vi "Write tsignal and tsensor elements u bazu_Core.vi"(9 "System_settings IN":T1={"Units in the system"=[], "dBase names by units"=[], "TCP/IP processing units addresses"=[], "TCP/IP server address"="", "dBase User Name_Cli"="codis_cli", "dBase User Password_Cli"="codis_cli", "dBase User Name_Med"="codis_med_wrt", "dBase User Password_Med"="codis_med_wrt", "Sampling rate [Hz]"=0.0, "FTP Server User name, cRIO"="", "FTP Server Password, cRIO"="", "OnScreenKeyboardPopUp"=FALSE, "Number of points to collect"=0, "Main Window has title bar?"=FALSE, "Demo?"=FALSE, "dBase - Limit # of  elements to read"=0, "dBase Backup"={"dBase Backup Base Folder"="c:\\codis\\backup\\", "Remote dBase Backup Configured?"=TRUE}, "System Status"={"System Monitor Refresh Rate (ms)"=10000, "System Status Log  File"="c:\\codis\\system_info.txt", "Max number of elements to read\n"=26611200}, "Number of points to average for stationary state"=[60], "Number of points to collect for saving waveforms per channel"=[60], "Sources per Unit"=[], "TCP/IP_client_mediator_communication ports"=2058, "TCP/IP processing_units _mediator_communication ports"=2055}, 10 "1D array of Pan Cluster IN":T10[](array[typedef]) {"Absolute Minimum Air Gap per Plane"."Absolute AG Minimum Pole Number" format="%.3f"; "Absolute Minimum Air Gap per Plane"."Absolute AG Minimum Value" format="%.3f"; "Magnetic Field Data"."Maximum by Pole Number" format="%.3f"; "Air Gap Data"."Minimum by Pole Number" format="%.3f"; "Orbit(s) - XY"."Orbit XY Graphs (Synthesized from Selected Harmonics and DC)"."?" format="%.3f"; "Orbit(s) - XY"."Orbit XY Graphs (Synthesized from Selected Harmonics and DC)"."?" format="%.3f"; "Orbit(s) - XY"."Orbit XY Graphs (Glided and Averaged on One Revolution)"."?" format="%.3f"; "Orbit(s) - XY"."Orbit XY Graphs (Glided and Averaged on One Revolution)"."?" format="%.3f"; "Orbit(s) - XY"."Orbit XY Graphs (Unaveraged)"."?" format="%.3f"; "Orbit(s) - XY"."Orbit XY Graphs (Unaveraged)"."?" format="%.3f"}, 11 "1D array of Waveform Cluster IN":T4[](array[typedef]) {"Analysis Parameters"."SP2Pmax"."Filter Parameters"."low cutoff freq: fl" format="%0.4f"; "Analysis Parameters"."SP2Pmax"."Filter Parameters"."high cutoff freq: fh" format="%0.2f"; "Analysis Parameters"."LoadAngleDelta"."Multiplication Factor" format="%.1f"; "Analysis Parameters"."LoadAngleDelta"."What harmonic? (for example 24th (48 pole machine))" format="%.1f"; "Analysis Parameters"."Peak2Peak"."Filter Parameters"."low cutoff freq: fl" format="%0.4f"; "Analysis Parameters"."Peak2Peak"."Filter Parameters"."high cutoff freq: fh" format="%0.2f"; "Analysis Parameters"."RMS"."Filter Parameters"."order" format="%0.4f"; "Analysis Parameters"."RMS"."Filter Parameters"."low cutoff freq: fl" format="%0.2f"; "Analysis Parameters"."RMS"."Filter Parameters"."high cutoff freq: fh" format="%0.2f"; "Analysis Parameters"."EqPeak"."Filter Parameters"."low cutoff freq: fl" format="%0.4f"; "Analysis Parameters"."EqPeak"."Filter Parameters"."high cutoff freq: fh" format="%0.2f"; "Analysis Parameters"."Peak"."Filter Parameters"."low cutoff freq: fl" format="%0.4f"; "Analysis Parameters"."Peak"."Filter Parameters"."high cutoff freq: fh" format="%0.2f"; "Analysis Parameters"."snPh"."What harmonic?" format="%.1f"; "Analysis Parameters"."snA"."Multiplication Factor" format="%.1f"; "Analysis Parameters"."snA"."What harmonic?" format="%.1f"; "Analysis Parameters"."Smax"."Filter Parameters"."low cutoff freq: fl" format="%0.4f"; "Analysis Parameters"."Smax"."Filter Parameters"."high cutoff freq: fh" format="%0.2f"; "Analysis Parameters"."RPM"."Signal Threshold" format="%.1f"}) -> (0 "error  OUT":errorcluster)   [LabVIEW 2014]
uses:
  common/typedefs/Pan_Cluster_Core.ctl
  common/typedefs/Condition_Vector_Cluster_Core.ctl
  common/typedefs/Unit_Names_Core.ctl
  common/typedefs/Data_Sources_Core.ctl
  common/typedefs/Waveforms_Cluster_Core.ctl
  common/typedefs/Types_of_Signals_Core.ctl
  common/typedefs/Types_of_Analyses_Core.ctl
  common/typedefs/Analysis_Parameters_Cluster_Core.ctl
  <vilib>/Analysis/3filter.llb/Filter Passband Type.ctl
  common/typedefs/Integration_Types_Core.ctl
  common/typedefs/System_Settings_Cluster_Client_Mediator_Core.ctl
  <vilib>/addons/database/Connection.llb/DB Tools Open Connec (String).vi
  <vilib>/addons/database/NI_Database_API.lvlib
  <vilib>/Analysis/NI_AALBase.lvlib
panel:
  out "error out 2":errorcluster
  out "error out":errorcluster
  out "Condition Vector Name":string[](array[string])
  out "Condition Vector Label":string[](array[string])
  out "Waveform Name":string[](array[string])
  out "Waveform Label":string[](array[string])
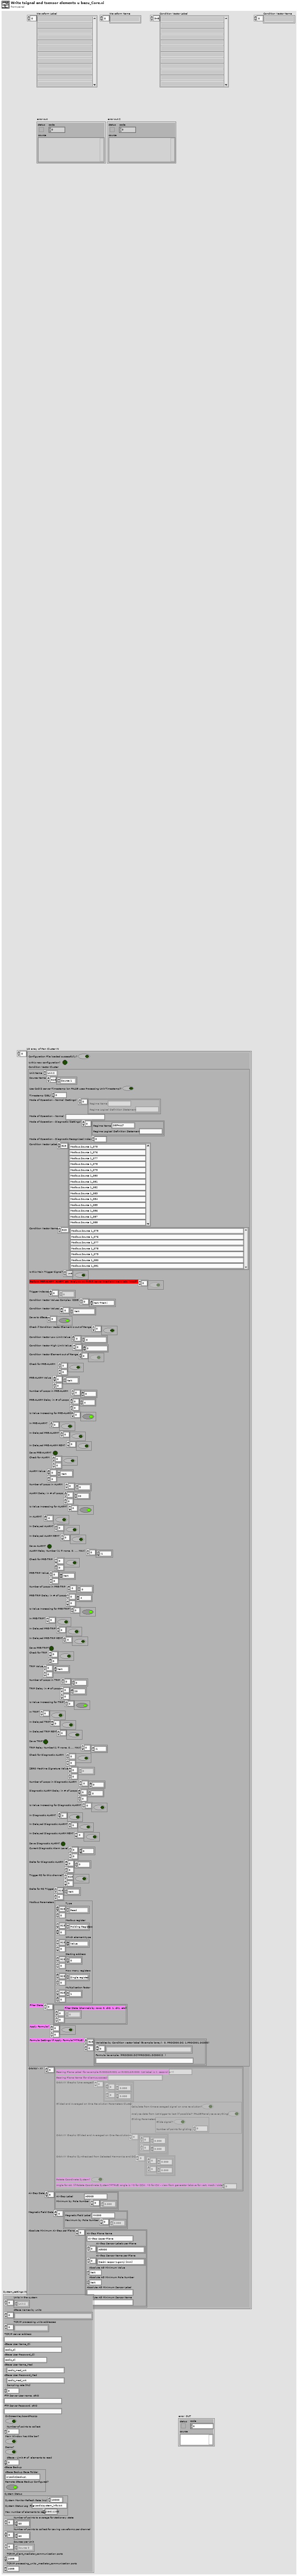
[diagram p1: front panel]
types:
  T1 = typedef "System_Settings_Cluster_Client_Mediator_Core.ctl" = cluster{"Units in the system":T2[], "dBase names by units":string[], "TCP/IP processing units addresses":string[], "TCP/IP server address":string, "dBase User Name_Cli":string, "dBase User Password_Cli":string, "dBase User Name_Med":string, "dBase User Password_Med":string, "Sampling rate [Hz]":dbl, "FTP Server User name, cRIO":string, "FTP Server Password, cRIO":string, "OnScreenKeyboardPopUp":bool, "Number of points to collect":u32, "Main Window has title bar?":bool, "Demo?":bool, "dBase - Limit # of  elements to read":u32, "dBase Backup":cluster{"dBase Backup Base Folder":string, "Remote dBase Backup Configured?":bool}, "System Status":cluster{"System Monitor Refresh Rate (ms)":u32, "System Status Log  File":string, "Max number of elements to read\n":i64}, "Number of points to average for stationary state":i32[], "Number of points to collect for saving waveforms per channel":i32[], "Sources per Unit":T3[], "TCP/IP_client_mediator_communication ports":u16, "TCP/IP processing_units _mediator_communication ports":u16}
  T2 = typedef "Unit_Names_Core.ctl" = enum16{"Not used", "Unit 1", "Unit 2", "Unit 3", "Unit 4", "Unit 5", "Unit 6", "Unit 7", "Unit 8", "Unit 9"}
  T3 = typedef "Data_Sources_Core.ctl" = enum16{"Not Used", "Source 0", "Source 1", "Source 2", "Source 3", "Source 4", "Source 5", "Source 6", "Source 7", "Source 8", "Source 9", "Source 10", "Source 11", "Source 12", "Source 13", "Source 14", "Source 15", "Source 16", "Source 17", "Source 18", "Source 19", "Source 20"}
  T4 = typedef "Waveforms_Cluster_Core.ctl" = cluster{"Configuration File loaded successfully? ":bool, "Is this new configuration?":bool, "Unit Name":T2, "Waveform Source":T3[], "Use CoDiS server Timestamp (on FALSE uses Processing Unit Timestamp)?":bool, "Sampling Rate [Hz]":u32[], "Timestamp (DBL)":dbl, "Mode of Operation - Normal":string, "Mode of Operation - Diagnostic":string, "Waveform Physical Channel":u16[], "Waveform Label":string[], "Waveform Name":string[], "Signal Type":cluster{"Signal Type":T5, "# of signal of particular type":u8}[], "Is this Main Trigger Signal?":bool[], "Slope":dbl[], "Intercept":dbl[], "Waveform Values":sgl[][], "Analyse?":bool[], "Save to database?":bool[], "Analyses to Perform":T6[][], "Perform this analysis on a CoDiS server?":bool[][], "General Parameters":cluster{"Number of Poles":u8, "Grid Frequency":sgl}, "Analysis Parameters":T7[][], "Save now to dBase?":bool, "Waveform Length for Saving [s]":u16, "Pretrigger Length when Saving Waveform [s]":u16, "Next Timestamp to autosave at (DBL)":dbl, "Description of Waveforms Events":string, "Event Type":string, "Save next RS event entirely? (on FALSE uses How many basic (acquisition) blocks of data (loops) to save?":bool, "Regime Name for which to save next RS event entirely":string, "Integration type":T9[], "Channel not OK?":bool[], "Channel Not OK?  Relay Number (-1 = none, 0, ..., MAX)":i16[], "Array of FPGA Filter Parameters":cluster{"Filter signal?":bool, "filter type":T8, "high cutoff freq: fh":dbl, "low cutoff freq: fl":dbl, "order":i32}[][], "Pre-Alarm Delay in Number of Loops ":u16, "Pre-Trip Delay in Number of Loops ":u16}
  T5 = typedef "Types_of_Signals_Core.ctl" = enum16{"Not Used", "Trigger (TRG???)", "Relative Vibrations (RV???)", "Absolute Vibrations (AV???)", "Air Gap (AG???)", "Magnetic Field (MX???)", "Voltage (VOL???)", "Current (CURR???)", "Process (PROC???)", "Cavitation (CAV???)", "Non Standard (NONST???)", "Axial Displacement (AXD???)", "Absolute Vibrations Stator Core (AVSC???)"}
  T6 = typedef "Types_of_Analyses_Core.ctl" = enum16{"Exit Analysis Loop", "Do Nothing", "RPM", "Smax", "SP2Pmax", "snA", "snPh", "Rest", "Peak", "EqPeak", "Peak2Peak", "RMS", "DC", "DC from Extrema", "Min Value", "Max Value", "Min Value by Pole", "Max Value by Pole", "Max Diff by Pole", "Max Diff Pole Number", "Min from Extrema", "Max from Extrema", "Active Power from DFT", "Active Power by Integration", "Reactive Power from DFT", "Reactive Power by Integration", "Apparent Power", "Ampl@Freq", "Phase Difference", "Load Angle Delta", "THD", "Signal Frequency", "Eta", "Non standard (CoDiS server - manual) 0", "Non standard (CoDiS server - manual) 1", "Non standard (CoDiS server - manual) 2", "Non standard (CoDiS server - manual) 3", "Non standard (CoDiS server - manual) 4", "Non standard (CoDiS server - manual) 5", "Non standard (CoDiS server - manual) 6", "Non standard (CoDiS server - manual) 7", "Non standard (CoDiS server - manual) 8", "Non standard (CoDiS server - manual) 9", "Non standard (CoDiS server - manual) 10", "Non standard (CoDiS server - manual) 11", "Non standard (CoDiS server - manual) 12", "Non standard (CoDiS server - manual) 13", "Non standard (CoDiS server - manual) 14", "Non standard (CoDiS server - manual) 15", "Non standard (CoDiS server - manual) 16", "Non standard (CoDiS server - manual) 17", "Non standard (CoDiS server - manual) 18", "Non standard (CoDiS server - manual) 19", "CosFi", "Total THD", "Crest Factor"}
  T7 = typedef "Analysis_Parameters_Cluster_Core.ctl" = cluster{"DC":cluster{"Analyze data from 1st trigger to last (if possible)? (FALSE=analyze everything)":bool}, "DCExtrema":cluster{"Calculate DC from all Pole Values":bool, "Poles to use in DC calculation (if Calculate DC from all Pole Values is FALSE)":u8[], "Condition Vector Label begin Part (MinPole or MaxPole)":string, "Addition to Condition Vector Label (example: 000)":string}, "RPM":cluster{"Signal Threshold":sgl, "Pulse Width (should be >= 2 depending on signal noise)":i32, "Trigger on rising edge? (FALSE=trigger on falling)":bool}, "Smax":cluster{"Combine with which Waveform Label? (for example: RV001)":string, "Calculate from time-averaged signal on one revolution?":bool, "Analyze data from 1st trigger to last (if possible)? (FALSE=analyze everything)":bool, "Filter Parameters":cluster{"Filter signal?":bool, "filter type":T8, "high cutoff freq: fh":dbl, "low cutoff freq: fl":dbl, "order":i32, "Process as ring-buffer signal?":bool}, "Gliding Parameters":cluster{"Glide signal?":bool, "Number of points for gliding":u16}, "Average all calculated values for Smax - if present (each revolution)? (FALSE=take absolute maximum)":bool, "Addition to Condition Vector Label (example: 000)":string}, "SP2Pmax":cluster{"Combine with which Waveform Label? (for example: RV001)":string, "Calculate from time-averaged signal on one revolution?":bool, "Analyze data from 1st trigger to last (if possible)? (FALSE=analyze everything)":bool, "Filter Parameters":cluster{"Filter signal?":bool, "filter type":T8, "high cutoff freq: fh":dbl, "low cutoff freq: fl":dbl, "order":i32, "Process as ring-buffer signal?":bool}, "Gliding Parameters":cluster{"Glide signal?":bool, "Number of points for gliding":u16}, "Average all calculated values for SP2Pmax - if present (each revolution)? (FALSE=take absolute maximum)":bool, "Addition to Condition Vector Label (example: 000)":string}, "snA":cluster{"What harmonic?":sgl, "Calculate Amplitude (TRUE) or RMS (FALSE)?":bool, "Multiplication Factor":sgl, "Calculate Amplitude for Air Gap type signals? (from MinPole Values)":bool}, "snPh":cluster{"What harmonic?":sgl}, "Peak":cluster{"Calculate from time-averaged signal (one-revolution)?":bool, "Analyze data from 1st trigger to last (if possible)? (FALSE=analyze everything)":bool, "Filter Parameters":cluster{"Filter signal?":bool, "filter type":T8, "high cutoff freq: fh":dbl, "low cutoff freq: fl":dbl, "order":i32, "Process as ring-buffer signal?":bool}, "Gliding Parameters":cluster{"Glide signal?":bool, "Number of points for gliding":u16}, "Average all calculated values for Peak - if present (each revolution)? (FALSE=take absolute maximum)":bool, "Addition to Condition Vector Label (example: 000)":string}, "Peak2Peak":cluster{"Calculate from time-averaged signal (one-revolution)?":bool, "Analyze data from 1st trigger to last (if possible)? (FALSE=analyze everything)":bool, "Gliding Parameters":cluster{"Glide signal?":bool, "Number of points for gliding":u16}, "Filter Parameters":cluster{"Filter signal?":bool, "filter type":T8, "high cutoff freq: fh":dbl, "low cutoff freq: fl":dbl, "order":i32, "Process as ring-buffer signal?":bool}, "Average all calculated values for Peak2Peak - if present (each revolution)? (FALSE=take absolute maximum)":bool, "Addition to Condition Vector Label (example: 000)":string}, "EqPeak":cluster{"Calculate from time-averaged signal (one-revolution)?":bool, "Analyze data from 1st trigger to last (if possible)? (FALSE=analyze everything)":bool, "Average all calculated values for EqPeak - if present (each revolution)? (FALSE=take absolute maximum)":bool, "Filter Parameters":cluster{"Filter signal?":bool, "filter type":T8, "high cutoff freq: fh":dbl, "low cutoff freq: fl":dbl, "order":i32, "Process as ring-buffer signal?":bool}, "Which Condition Vector Label addition to use for RMS (example: 001)":string, "Addition to Condition Vector Label (example: 000)":string}, "RMS":cluster{"Calculate from time-averaged signal (one-revolution)?":bool, "Analyze data from 1st trigger to last (if possible)? (FALSE=analyze everything)":bool, "Subtract DC before RMS calculation?":bool, "Filter Parameters":cluster{"Filter signal?":bool, "filter type":T8, "high cutoff freq: fh":dbl, "low cutoff freq: fl":dbl, "order":i32, "Process as ring-buffer signal?":bool}, "Gliding Parameters":cluster{"Glide signal?":bool, "Number of points for gliding":u16}, "Average all calculated values for RMS - if present (each revolution)? (FALSE=take absolute maximum)":bool, "Addition to Condition Vector Label (example: 000)":string}, "Rest":cluster{"Calculate from all calculated harmonics?":bool, "Condition Vector Label to use for substraction (if Calculate from all calculated harmonics?=FALSE)":string[], "Calculate by subtracting from EqPeak Value? (FALSE=calculate by subtracting from RMS Value)":bool, "Which Condition Vector Label addition to use for EqPeak (example: 001)":string, "Addition to Condition Vector Label (example: 000)":string}, "MinByPole":cluster{"First Pole Number after Trigger (indexes correspond to Normal regime settings)":u8[], "Are Pole Numbers in ascending order in time?  (indexes correspond to Normal regime settings)":bool[], "Average all calculated values for that Pole? (FALSE=take absolute minimum)":bool, "Coerce Upper Limit":sgl, "Compensate 1st harmonic in waveform?":bool}, "MinExtrema":cluster{"Calculate Min Extrema from all Pole Values":bool, "Poles to use in Min Extrema calculation (if Calculate Min Extrema from all Pole Values is FALSE)":u8[], "Condition Vector Label begin Part (MinPole or MaxPole)":string}, "MaxByPole":cluster{"First Pole Number after Trigger (indexes correspond to Normal regime settings)":u8[], "Are Pole Numbers in ascending order in time? (indexes correspond to Normal regime settings)":bool[], "Average all calculated values for that Pole? (FALSE=take absolute maximum)":bool, "Calculate with abs(Signal)?":bool, "Subtract DC before calculation?":bool, "Coerce Lower Limit":sgl}, "MaxExtrema":cluster{"Calculate Max Extrema from all Pole Values":bool, "Poles to use in Max Extrema calculation (if Calculate Max Extrema from all Pole Values is FALSE)":u8[], "Condition Vector Label begin Part (MinPole or MaxPole)":string}, "MaxDiffByPole":cluster{"First Pole Number after Trigger (indexes correspond to Normal regime settings)":u8[], "Are Pole Numbers in ascending order in time? (indexes correspond to Normal regime settings)":bool[], "Condition Vector Label begin Part (MinPole or MaxPole)":string}, "Min":cluster{"Analyze data from 1st trigger to last (if possible)? (FALSE=analyze everything)":bool, "Calculate from time-averaged signal on one revolution?":bool, "Gliding Parameters":cluster{"Glide signal?":bool, "Number of points for gliding":u16}, "Average all calculated values for Min - if present (each revolution)? (FALSE=take absolute maximum)":bool}, "Max":cluster{"Analyze data from 1st trigger to last (if possible)? (FALSE=analyze everything)":bool, "Calculate from time-averaged signal on one revolution?":bool, "Gliding Parameters":cluster{"Glide signal?":bool, "Number of points for gliding":u16}, "Average all calculated values for Max - if present (each revolution)? (FALSE=take absolute maximum)":bool}, "ActivePower":cluster{"Calculate from Phase Voltages and Currents?":bool, "Phase Voltage Condition Vector Label (R, S, T) (for example: VOL000.s24.00A, VOL001.s24.00A, VOL002.s24.00A)":string[], "Phase Current Condition Vector Label (R, S, T) (for example: CURR000.s24.00A, CURR001.s24.00A, CURR002.s24.00A)":string[]}, "ReactivePower":cluster{"Calculate from Phase Voltages and Currents?":bool, "Phase Voltage Condition Vector Label (R, S, T) (for example: VOL000.s24.00A, VOL001.s24.00A, VOL002.s24.00A)":string[], "Phase Current Condition Vector Label (R, S, T) (for example: CURR000.s24.00A, CURR001.s24.00A, CURR002.s24.00A)":string[]}, "LoadAngleDelta":cluster{"What harmonic? (for example 24th (48 pole machine))":sgl, "Delta0":sgl, "Which Voltage Waveform Label? (for example: VOL000)":string, "Combine (multiply) with which Air Gap Waveform Label? (for example: AG000)":string, "Multiplication Factor":sgl}, "ActivePowerByIntegration":cluster{"Phase Voltage Waveform Labels (R,S,T)":string[], "Phase Current Waveform Labels (R,S,T)":string[], "Analyze data from 1st trigger to last (if possible)? (FALSE=analyze everything)":bool}, "RectivePowerByIntegration":cluster{"Phase Voltage Waveform Vector Labels (R,S,T)":string[], "Phase Current Waveform Labels (R,S,T)":string[], "System Electric Frequency [Hz]":sgl, "Analyze data from 1st trigger to last (if possible)? (FALSE=analyze everything)":bool}, "Ampl@Freq":cluster{"Frequency [Hz]":sgl, "Calculate Amplitude? (FALSE=calculate RMS)":bool}, "PhaseDifference":cluster{"Combine with which Waveform Label?":string}, "CosFi":cluster{"Voltage Waveform Labels (R,S,T)":string[], "Current Waveform Labels (R,S,T)":string[]}, "Total THD":cluster{"THD Condition Vector Label (R, S, T) (for example: VOL000.THD, VOL001.THD, VOL002.THD)":string[]}, "Crest Factor":cluster{"Addition to Condition Vector Label (example: 000)":string, "Which Condition Vector Label addition to use for Peak (example: 001)":string, "Which Condition Vector Label addition to use for RMS (example: 001)":string}}
  T8 = typedef "NI_AALBase.lvlib/Filter Passband Type.ctl" = enum32{"Lowpass", "Highpass", "Bandpass", "Bandstop"}
  T9 = typedef "Integration_Types_Core.ctl" = enum16{"Do not integrate", "Integrate once", "Integrate twice"}
  T10 = typedef "Pan_Cluster_Core.ctl" = cluster{"Configuration File loaded successfully?":bool, "Is this new configuration?":bool, "Condition Vector Cluster":T11, "Orbit(s) - XY":cluster{"Bearing Plane Label (for example RV000&RV001 or RV001&RV000; 1st label is X, second is Y)":string, "Bearing Plane Name (for client purposes)":string, "Orbit XY Graphs (Unaveraged)":cluster{sgl[], sgl[]}[], "Glided and Averaged on One Revolution Parameters Cluster":cluster{"Calculate from time-averaged signal on one revolution?":bool, "Analyze data from 1st trigger to last (if possible)? (FALSE=analyze everything)":bool, "Gliding Parameters":cluster{"Glide signal?":bool, "Number of points for gliding":u16}}, "Orbit XY Graphs (Glided and Averaged on One Revolution)":cluster{sgl[], sgl[]}[], "Orbit XY Graphs (Synthesized from Selected Harmonics and DC)":cluster{sgl[], sgl[]}[], "Rotate Coordinate System?":bool, "Angle for rot. (if Rotate Coordinate System?=TRUE; angle is >0 for CCW, <0 for CW - view from generator (above for vert. mach.) side)":sgl}[], "Air Gap Data":cluster{"Air Gap Label":string, "Minimum by Pole Number":sgl[]}[], "Magnetic Field Data":cluster{"Magnetic Field Label":string, "Maximum by Pole Number":sgl[]}[], "Absolute Minimum Air Gap per Plane":cluster{"Air Gap Plane Name":string, "Air Gap Sensor Labels per Plane":string[], "Air Gap Sensor Name per Plane":string[], "Absolute AG Minimum Value":sgl, "Absolute AG Minimum Pole Number":sgl, "Absolute AG Minimum Sensor Label":string, "Absolute AG Minimum Sensor Name":string}[]}
  T11 = typedef "Condition_Vector_Cluster_Core.ctl" = cluster{"Unit Name":T2, "Source Name":T3[], "Use CoDiS server Timestamp (on FALSE uses Processing Unit Timestamp)?":bool, "Timestamp (DBL)":dbl, "Mode of Operation - Normal (Settings)":cluster{"Regime Name":string, "Regime Logical Definition Statement":string}[], "Mode of Operation - Normal":string, "Mode of Operation - Diagnostic (Settings)":cluster{"Regime Name":string, "Regime Logical Definition Statement":string}[], "Mode of Operation - Diagnostic Recognized Index":i16, "Condition Vector Label":string[], "Condition Vector Name":string[], "Is this Main Trigger Signal?":bool[], "Perform PRE-ALARM, ALARM, etc. Analysis on CoDiS server (mediator main calc. loop)?":bool[], "Trigger Indexes":u32[], "Condition Vector Values Complex (CDB)":cdb[], "Condition Vector Values":sgl[], "Save to dBase":bool[], "Check if Condition Vector Element is out of Range":bool[], "Condition Vector Low Limit Value":sgl[], "Condition Vector High Limit Value":sgl[], "Condition Vector Element out of Range":bool[], "Check for PRE-ALARM":bool[][], "PRE-ALARM Value":sgl[][], "Number of Loops in PRE-ALARM":u32[], "PRE-ALARM Delay in # of Loops":u16[][], "Is Value Increasing for PRE-ALARM?":bool[], "In PRE-ALARM?":bool[], "In Delayed PRE-ALARM?":bool[], "In Delayed PRE-ALARM REM?":bool[], "Save PRE-ALARM?":bool, "Check for ALARM":bool[][], "ALARM Value":sgl[][], "Number of Loops in ALARM":u32[], "ALARM Delay in # of Loops":u16[][], "Is Value Increasing for ALARM?":bool[], "In ALARM?":bool[], "In Delayed ALARM?":bool[], "In Delayed ALARM REM?":bool[], "Save ALARM?":bool, "ALARM Relay Number (-1 = none, 0, ..., MAX)":i16[], "Check for PRE-TRIP":bool[][], "PRE-TRIP Value":sgl[][], "Number of Loops in PRE-TRIP":u32[], "PRE-TRIP Delay in # of Loops":u16[][], "Is Value Increasing for PRE-TRIP?":bool[], "In PRE-TRIP?":bool[], "In Delayed PRE-TRIP?":bool[], "In Delayed PRE-TRIP REM?":bool[], "Save PRE-TRIP?":bool, "Check for TRIP":bool[][], "TRIP Value":sgl[][], "Number of Loops in TRIP":u32[], "TRIP Delay in # of Loops":u16[][], "Is Value Increasing for TRIP?":bool[], "In TRIP?":bool[], "In Delayed TRIP?":bool[], "In Delayed TRIP REM?":bool[], "Save TRIP?":bool, "TRIP Relay Number(-1 = none, 0,..., MAX)":i16[], "Check for Diagnostic ALARM":bool[][], "ZERO Machine Signature Value":dbl[][], "Number of Loops in Diagnostic ALARM":u32[], "Diagnostic ALARM Delay in # of Loops":u16[][], "Is Value Increasing for Diagnostic ALARM?":bool[], "In Diagnostic ALARM?":bool[], "In Delayed Diagnostic ALARM?":bool[], "In Delayed Diagnostic ALARM REM?":bool[], "Save Diagnostic ALARM?":bool, "Current Diagnostic Alarm Level":sgl[][], "Delta for Diagnostic ALARM":sgl[][], "Trigger RS for this channel?":bool[][], "Delta for RS Trigger":sgl[][], "Modbus Parameters":cluster{"Type":enum16{"Read", "Write", "None"}[][], "Modbus register":enum16{"Coils", "Discrete Inputs", "Input Registers", "Holding Registers"}[][], "Which element type":enum16{"Value", "Alarm", "Trip"}[][], "Starting address":u16[][], "How many registers":enum16{"Single register", "HI-LO", "LO-HI"}[][], "Multiplication factor":dbl[][]}, "Filter State":cluster{"Filter State (channels by rows: 0. ch0, 1. ch1, etc))":dbl[][]}[], "Apply Formula?":bool[][], "Formula Settings (If Apply Formula?=TRUE)":cluster{"Variables by Condition vector label (Example (array):  0. PROC000.DC; 1.PROC001.DC000)":string[], "Formula (example: (PROC000.DC+PROC001.DC000)/2  )":string}[][]}
  T12 = typedef "NI_Database_API.lvlib/Conn ObjectReference.ctl" = refnum<k1>
  T13 = cluster{i32, "String":string, "String":string, "String":string}
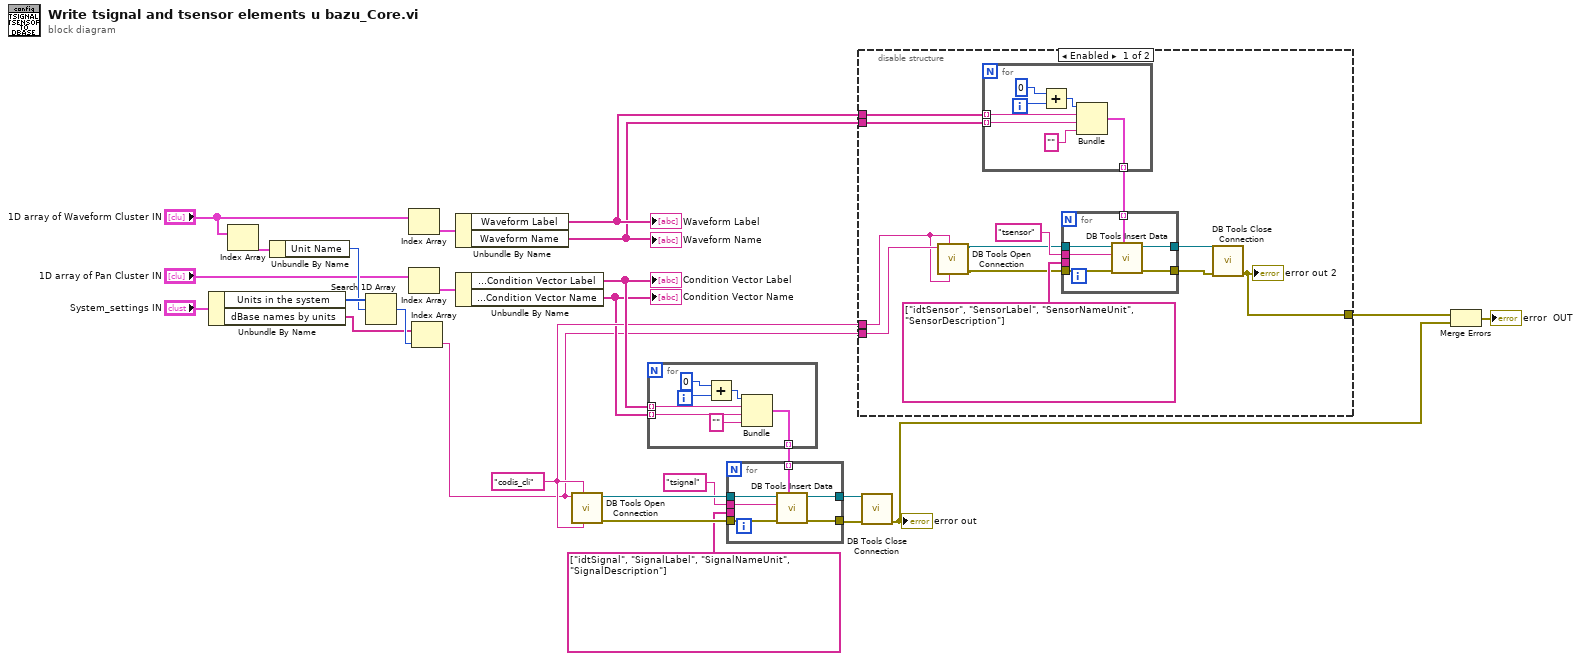
[diagram p0: block diagram]
diagram:
  w17 = "codis_cli" ("userID")
  n1 = Unbundle By Name("System_settings IN") -> ("Units in the system"=w10:T2[], "dBase names by units"=w8:string[])
  n2 = Index Array(array="1D array of Waveform Cluster IN") -> (element=w11:T4)  [unwired: 1 in]
  n3 = Unbundle By Name(w11) -> ("Unit Name"=w9:T2)
  n4 = Search 1D Array(1D array=w10, element=w9) -> (index of element=w12:i32)  [unwired: 1 in]
  n5 = Index Array(array="1D array of Waveform Cluster IN") -> (element=w15:T4)  [unwired: 1 in]
  n6 = Index Array(array="1D array of Pan Cluster IN") -> (element=w14:T10)  [unwired: 1 in]
  n7 = Index Array(array=w8, index=w12) -> (element=w7:string)
  n8 = Unbundle By Name(w15) -> ("Waveform Label"=w18:string[], "Waveform Name"=w16:string[])
  "Waveform Label" <- w18
  "Waveform Name" <- w16
  n9 = Unbundle By Name(w14) -> ("Condition Vector Cluster.Condition Vector Label"=w19:string[], "Condition Vector Cluster.Condition Vector Name"=w13:string[])
  "Condition Vector Label" <- w19
  "Condition Vector Name" <- w13
  n10 = call-poly <vilib>:"DB Tools Open Connection.vi"("password"=w17, "userID"=w17, "connection information"=w7) -> ("error out"=w25:errorcluster, "connection reference"=w26:T12)  [unwired: 5 in]
  n11 = for {
    tunnel: w19 -> [w33] mode=indexing
    tunnel: [w31] -> w23 mode=indexing
    tunnel: w13 -> [w27] mode=indexing
    i -> [w30]
    n12 = Add(x=0, y=w30) -> (x+y=w28:i32)
    n13 = Bundle(w28, "String"=w33, "String"=w27, "String"="") -> (w31:T13)  [unwired: 1 in]
  }
  n14 = for {
    tunnel: w26 -> [w39]
    tunnel: w25 -> [w38]
    tunnel: "tsignal" ("table") -> [w37]
    tunnel: w23 -> [w36] mode=indexing
    tunnel: [w35] -> w20
    tunnel: [w34] -> w21
    tunnel: string[] ["idtSignal", "SignalLabel", "SignalNameUnit", "SignalDescription"] ("columns") -> [_]
    n15 = call <vilib>:"DB Tools Insert Data.vi"("data"=w36, "error in (no error)"=w38, "table"=w37, "connection reference"=w39) -> ("error out"=w35:errorcluster, "connection reference out"=w34:T12)  [unwired: 6 in]
  }
  n16 = disable-structure shown="Enabled" {
    disable-tunnel: w18 -> [w47 _]
    disable-tunnel: w7 -> [w43 _]
    disable-tunnel: w17 -> [w42 _]
    disable-tunnel: w16 -> [w41 _]
    disable-tunnel: [w40 _] -> w3
    frame Enabled {
      n17 = call-poly <vilib>:"DB Tools Open Connection.vi"("password"=w42, "userID"=w42, "connection information"=w43) -> ("error out"=w48:errorcluster, "connection reference"=w49:T12)  [unwired: 5 in]
      n18 = for {
        tunnel: w47 -> [w58] mode=indexing
        tunnel: [w56] -> w46 mode=indexing
        tunnel: w41 -> [w52] mode=indexing
        i -> [w55]
        n19 = Add(x=0, y=w55) -> (x+y=w53:i32)
        n20 = Bundle(w53, "String"=w58, "String"=w52, "String"="") -> (w56:T13)  [unwired: 1 in]
      }
      n21 = for {
        tunnel: w49 -> [w64]
        tunnel: w48 -> [w63]
        tunnel: "tsensor" ("table") -> [w62]
        tunnel: w46 -> [w61] mode=indexing
        tunnel: [w60] -> w44
        tunnel: [w59] -> w45
        tunnel: string[] ["idtSensor", "SensorLabel", "SensorNameUnit", "SensorDescription"] ("columns") -> [_]
        n22 = call <vilib>:"DB Tools Insert Data.vi"("data"=w61, "error in (no error)"=w63, "table"=w62, "connection reference"=w64) -> ("error out"=w60:errorcluster, "connection reference out"=w59:T12)  [unwired: 6 in]
      }
      n23 = call <vilib>:"DB Tools Close Connection.vi"("error in (no error)"=w44, "connection reference"=w45) -> ("error out"=w40:errorcluster)  [unwired: 5 in]
      "error out 2" <- w40
    }
    frame Disabled {
    }
  }
  n24 = call <vilib>:"DB Tools Close Connection.vi"("error in (no error)"=w20, "connection reference"=w21) -> ("error out"=w2:errorcluster)  [unwired: 5 in]
  "error out" <- w2
  n25 = Merge Errors(w3, w2) -> (→"error  OUT":errorcluster)
